vi "Simple UDP - Receiver - 副本.vi"() -> ()   [LabVIEW 2020]
doc: "UDP协议与TCP的区别在于UDP不包括发送数据包信息的错误检查，因此无法保证接收端是否已接收所发数据。\n\nUDP可用于“广播”数据至整个网络，只需指定可包括全部的IP地址(255.255.255.255)以便发送信息至整个网络。 由于路由器或其他网络硬件通常拒绝转发超过一定点的数据，在实际应用中广播范围可能存在限制。"
panel:
  out "地址":u32
  out "波形图表 6":waveform(i32)[](graph)
  out "元素":i32[][](array[numeric])
  in  "停止 2":bool
  out "波形图表 5":i32[](graph)
  # "概述：演示使用UDP函数通过UDP连接接收数据。\n操作步骤：\n1.确保已运行Simple UDP - Sender.vi。\n2.运行VI。\n3.单击停止按钮停止VI。"
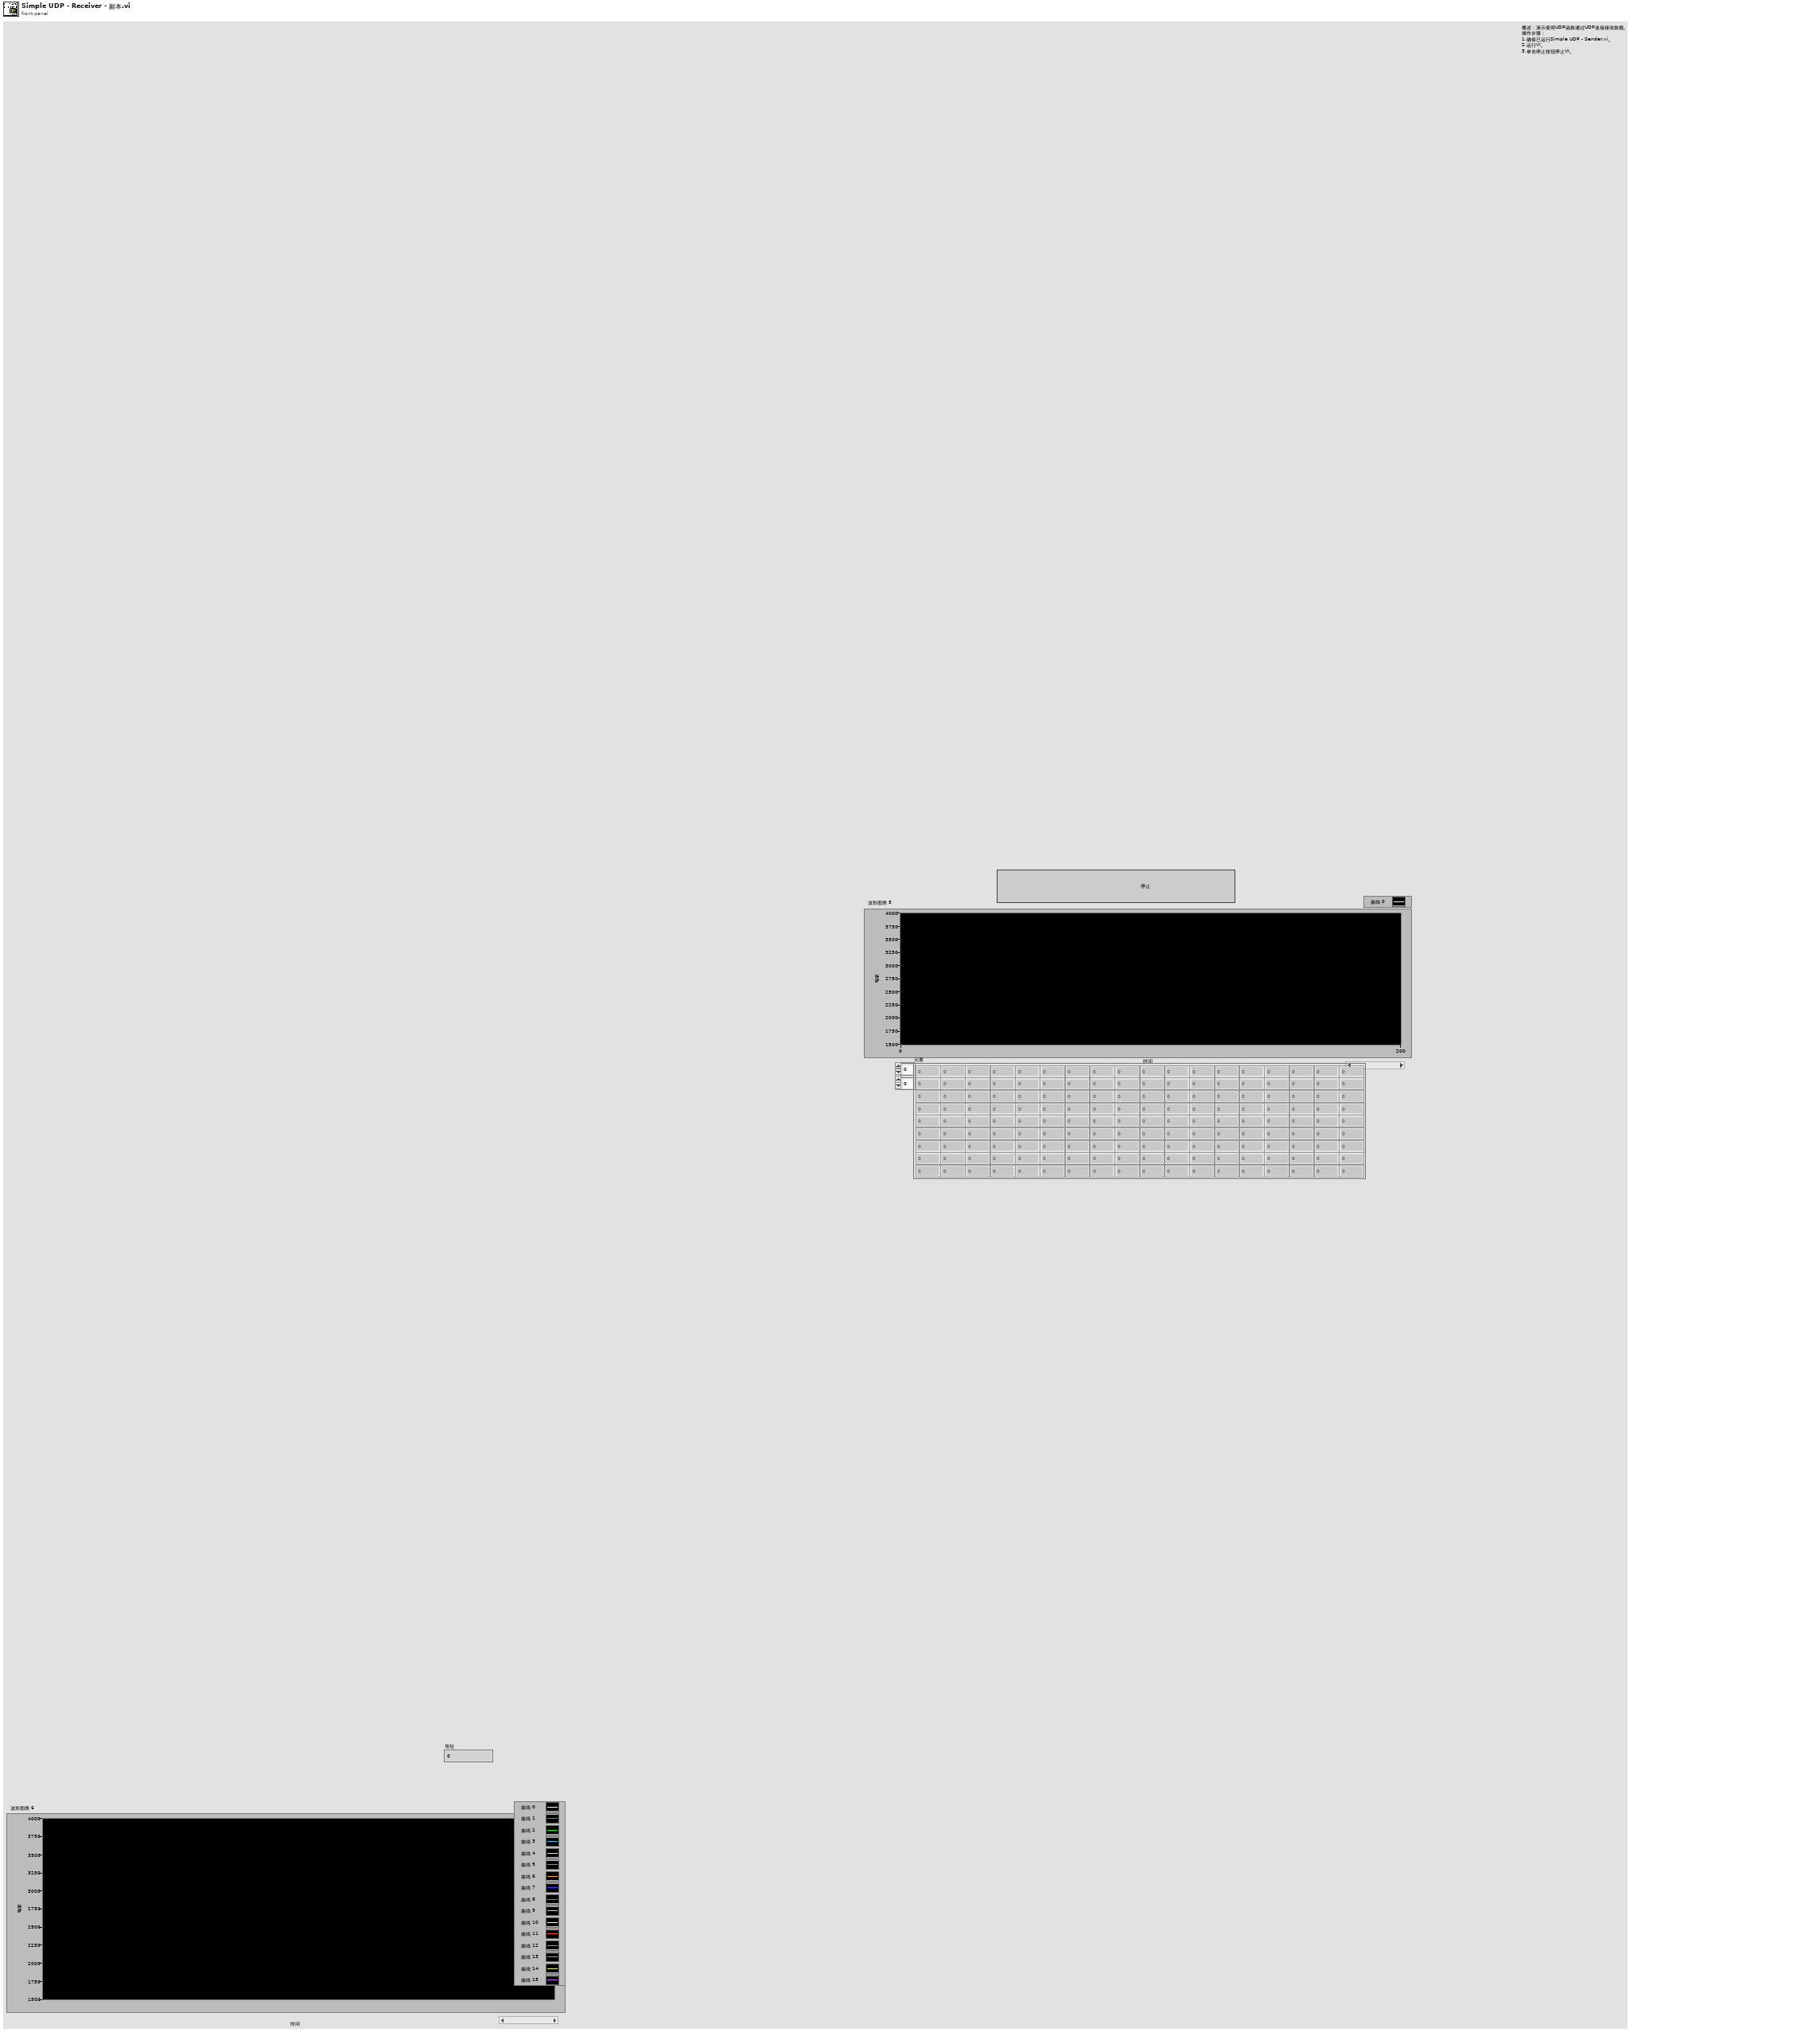
[diagram p1: front panel]
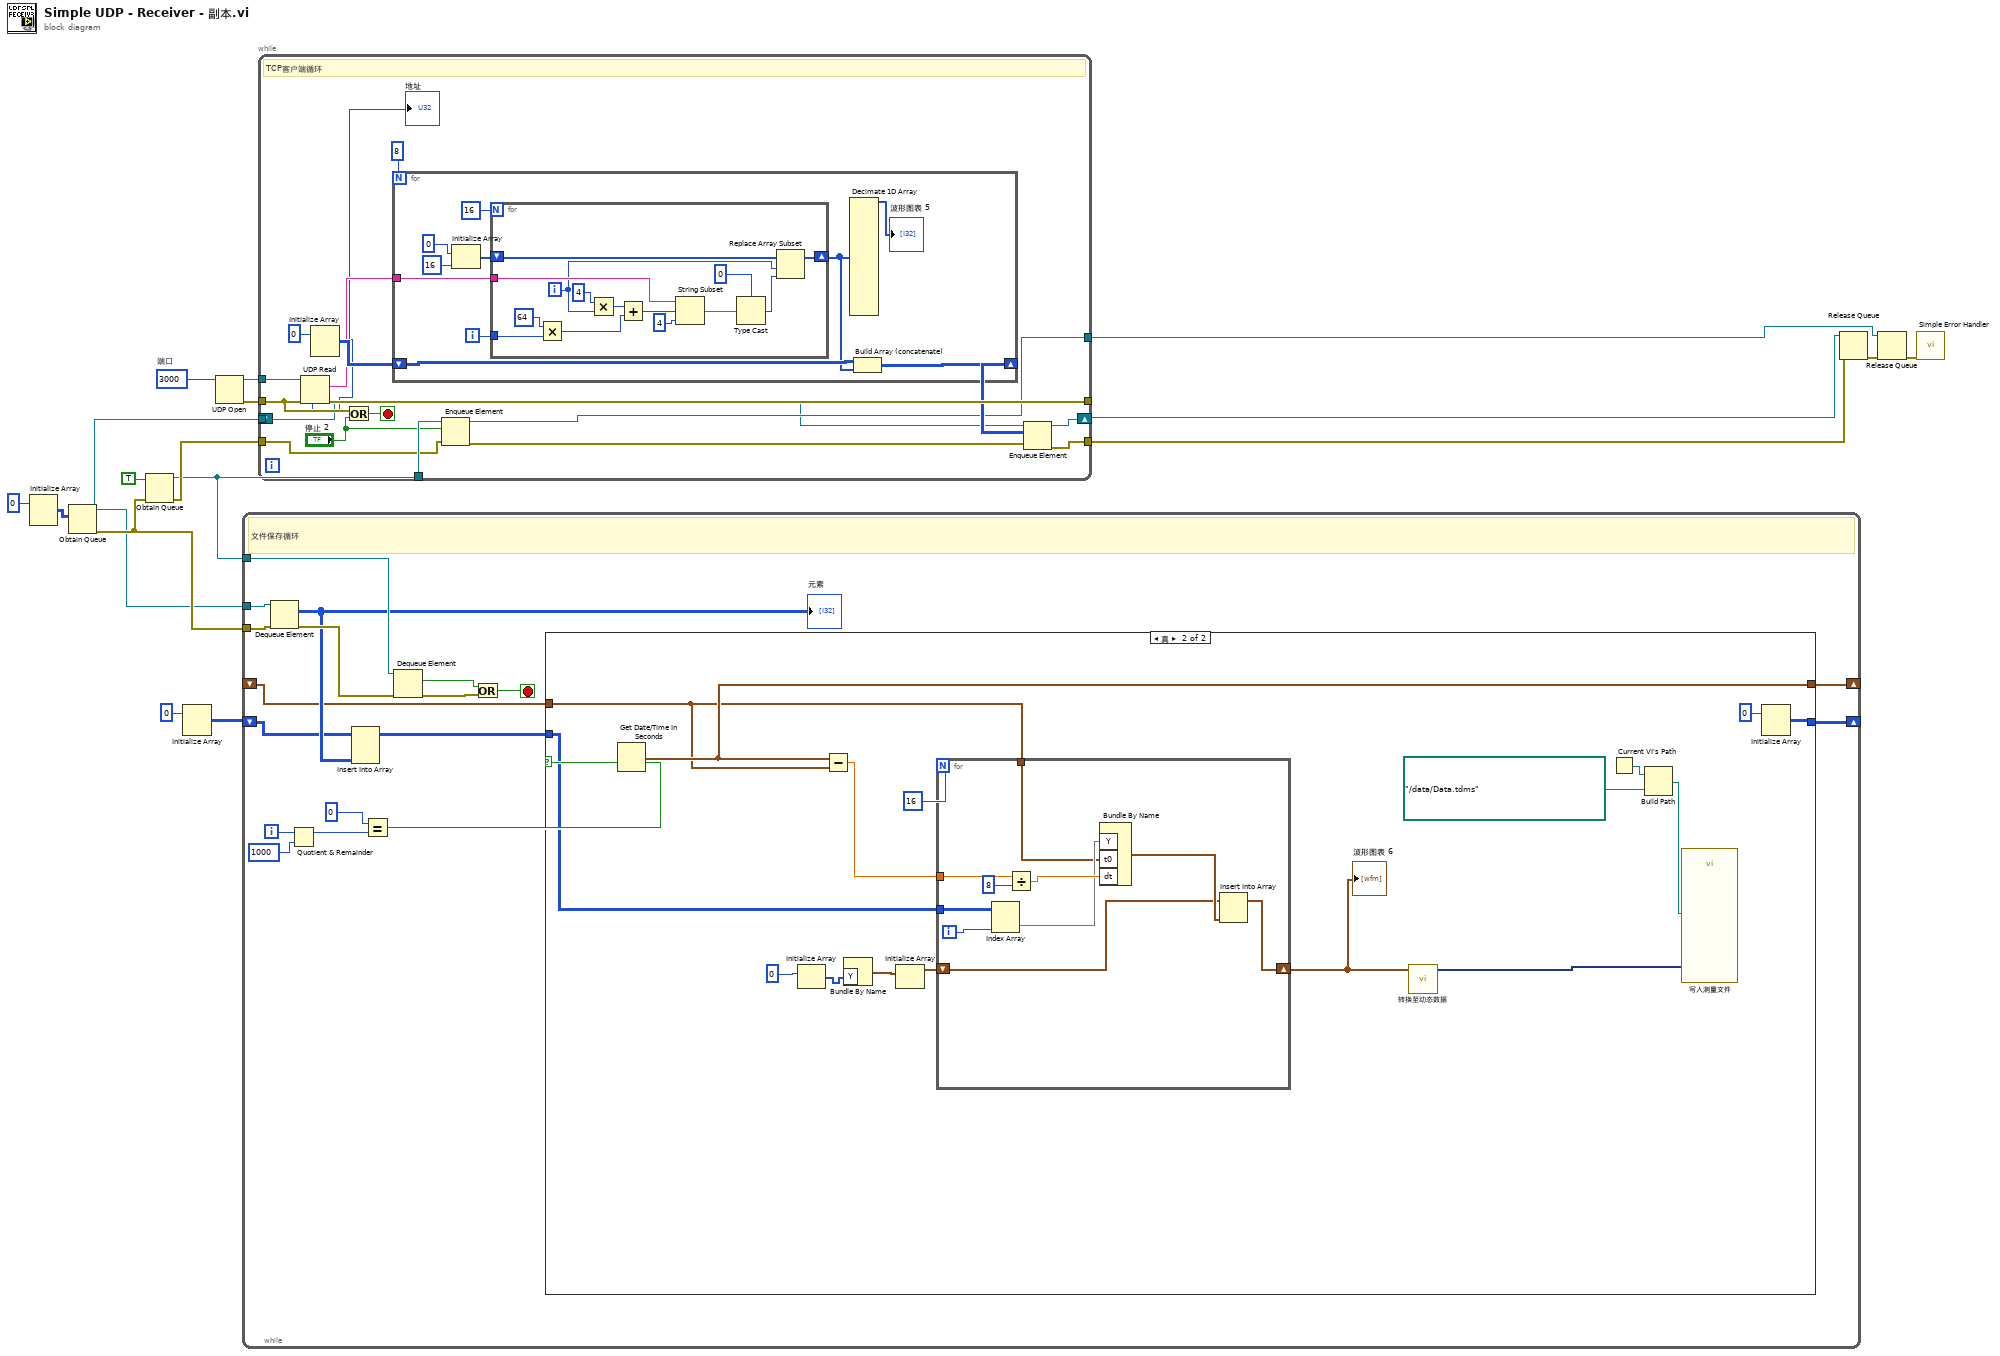
[diagram p0: block diagram]
diagram:
  w14 = u16 3000  # 端口
  n1 = Initialize Array(0) -> (w12:i32[][])  [unwired: 2 in]
  n2 = Obtain Queue(element data type=w12) -> (queue out=w6:refnum<queue>, error out=w7:errorcluster)  [unwired: 4 in, 1 out]
  n3 = Obtain Queue(element data type=TRUE, error in (no error)=w7) -> (queue out=w5:refnum<queue>, error out=w11:errorcluster)  [unwired: 3 in, 1 out]
  n4 = Initialize Array(0) -> (w1:i32[][])  [unwired: 2 in]
  n5 = UDP Open(11:w14) -> (port=w16:refnum<k16>, 0:w15:errorcluster)  [unwired: 4 in, 1 out]
  n6 = while {
    tunnel: w7 -> [w35]
    tunnel: w6 -> [w33]
    tunnel: w5 -> [w31]
    shift-right: [w20] -> _
    shift-left: w1 -> [w27]
    shift-right: [w19] -> _
    shift-left: _ -> [w18]
    i -> [w26]
    stop <- w34 stop-if-true
    # "文件保存循环"
    n7 = Dequeue Element(queue=w33, error in (no error)=w35) -> (element=w28:i32[][], error out=w32:errorcluster)  [unwired: 1 in, 2 out]
    "元素" <- w28
    n8 = Quotient & Remainder(x=w26, y=1000) -> (x-y*floor(x/y)=w23:i32)  [unwired: 1 out]
    n9 = Insert Into Array(array=w27, new element=w28) -> (w21:i32[][])  [unwired: 2 in]
    n10 = Equal?(x=0, y=w23) -> (x = y?=w22:bool)
    n11 = Dequeue Element(queue=w31, error in (no error)=w32) -> (element=w30:bool, error out=w29:errorcluster)  [unwired: 1 in, 2 out]
    n12 = Or(x=w30, y=w29) -> (x .or. y?=w34:bool)
    n13 = case shown="真" w22 {
      tunnel: w21 -> [w37 w43]
      tunnel: [w37 w52] -> w20
      tunnel: [w36 w42] -> w19
      tunnel: w18 -> [w36 w41]
      frame False {
      }
      frame True {
        n14 = Get Date/Time In Seconds() -> (seconds since 1Jan1904=w42:timestamp)
        n15 = Initialize Array(0) -> (w47:i32[])  [unwired: 1 in]
        n16 = Subtract(x=w42, y=w41) -> (x-y=w46:dbl)
        n17 = Bundle By Name ("创建波形")("Y"=w47) -> (w49:waveform(i32))  [unwired: 1 in]
        n18 = Initialize Array(w49) -> (w50:waveform(i32)[])  [unwired: 1 in]
        n19 = for {
          N: 16 -> [_]
          shift-right: [w61] -> w45
          shift-left: w50 -> [w60]
          tunnel: w46 -> [w59]
          tunnel: w43 -> [w56]
          tunnel: w41 -> [w54]
          i -> [w63]
          n20 = Index Array(array=w56, index (col)=w63) -> (element=w55:i32[])  [unwired: 1 in]
          n21 = Divide(x=w59, y=8) -> (x/y=w58:dbl)
          n22 = Bundle By Name ("创建波形")("Y"=w55, "t0"=w54, "dt"=w58) -> (w62:waveform(i32))  [unwired: 1 in]
          n23 = Insert Into Array(array=w60, new element=w62) -> (w61:waveform(i32)[])  [unwired: 1 in]
        }
        "波形图表 6" <- w45
        n24 = call "转换至动态数据"("Array of Waveforms"=w45) -> ("Dynamic Data Type"=w44:dynamicdata)  [unwired: 3 in]
        n25 = Current VI's Path() -> (path=w40:path)
        n26 = Build Path(base path=w40, name or relative path=path "../data/Data.tdms" ("file path")) -> (appended path=w38:path)
        n27 = call "写入测量文件"("Signals"=w44, "Filename"=w38) -> ()  [unwired: 15 in, 3 out]
        n28 = Initialize Array(0) -> (w52:i32[][])  [unwired: 2 in]
      }
    }
  }
  n29 = while {
    tunnel: w15 -> [w76]
    tunnel: w16 -> [w75]
    tunnel: [w77] -> _
    tunnel: w5 -> [w73]
    tunnel: [w68] -> w8
    tunnel: w6 -> [w65]
    tunnel: w11 -> [w71]
    tunnel: [w66] -> w3
    shift-right: [w67] -> w4
    shift-left: _ -> [_]
    stop <- w79 stop-if-true
    # "TCP客户端循环"
    n30 = UDP Read(connection ID=w75, 8:w76) -> (data out=w78:string, error out=w77:errorcluster, 6:→"地址":u32)  [unwired: 1 in, 3 out]
    n31 = Initialize Array(0) -> (w80:i32[][])  [unwired: 2 in]
    n32 = Or(x=w76, y="停止 2") -> (x .or. y?=w79:bool)
    n33 = for {
      N: u16 8 -> [_]
      tunnel: w78 -> [w91]
      shift-right: [w84] -> w69
      shift-left: w80 -> [w85]
      i -> [w86]
      n34 = Initialize Array(0, 16) -> (w87:i32[])
      n35 = for {
        N: i8 16 -> [_]
        tunnel: w91 -> [w103]
        tunnel: w86 -> [w99]
        shift-right: [w92] -> w82
        shift-left: w87 -> [w93]
        i -> [w94]
        n36 = Multiply(x=i8 64, y=w99) -> (x*y=w98:i32)
        n37 = Multiply(x=i8 4, y=w94) -> (x*y=w96:i32)
        n38 = Add(x=w96, y=w98) -> (x+y=w97:i32)
        n39 = String Subset(string=w103, offset (0)=w97, length (rest)=i8 4) -> (substring=w105:string)
        n40 = Type Cast(type=0, x=w105) -> (*(type *) &x=w95:i32)
        n41 = Replace Array Subset(array=w93, new element=w95, index=w94) -> (w92:i32[])
      }
      n42 = Decimate 1D Array(w82) -> (→"波形图表 5":i32[])  [unwired: 15 out]
      n43 = Build Array (concatenate)(w85, w82) -> (w84:i32[][])
    }
    n44 = Enqueue Element(queue=w73, element="停止 2", error in (no error)=w71) -> (queue out=w68:refnum<queue>, error out=w70:errorcluster)  [unwired: 1 in, 1 out]
    n45 = Enqueue Element(queue=w65, element=w69, error in (no error)=w70) -> (queue out=w67:refnum<queue>, error out=w66:errorcluster)  [unwired: 1 in, 1 out]
  }
  n46 = Release Queue(queue=w4, error in (no error)=w3) -> (error out=w10:errorcluster)  [unwired: 1 in, 2 out]
  n47 = Release Queue(queue=w8, error in (no error)=w10) -> (error out=w9:errorcluster)  [unwired: 1 in, 2 out]
  n48 = call <vilib>:"Simple Error Handler.vi"("error in (no error)"=w9) -> ()  [unwired: 4 in, 5 out]
